vi "TDMSLoader.vi"(8 "Error in":errorcluster, 11 "Measurements path":path=path "") -> (0 "Error out":errorcluster)   [LabVIEW 2019]
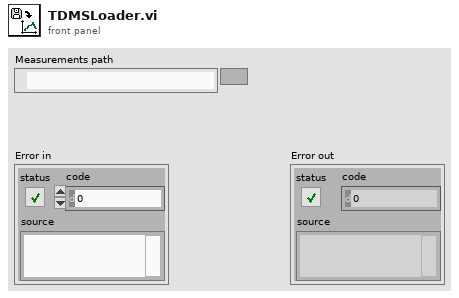
[diagram p1: front panel]
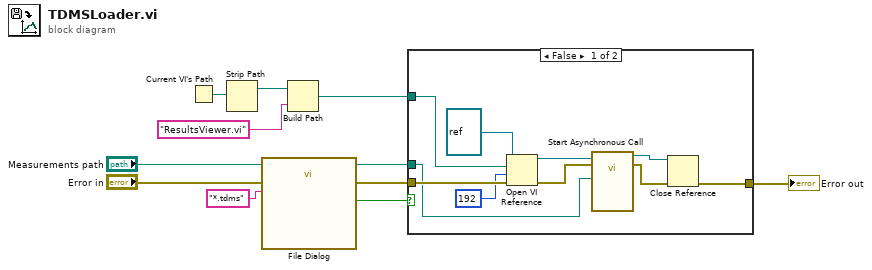
[diagram p0: block diagram]
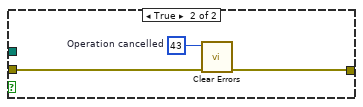
[diagram p2: hidden frame]
diagram:
  n1 = Current VI's Path() -> (path=w4:path)
  n2 = Strip Path(path=w4) -> (stripped path=w3:path)  [unwired: 1 out]
  n3 = call "File Dialog"("start path"="Measurements path", "error in"="Error in", "pattern (all files)"="*.tdms") -> ("selected path"=w10:path, "cancelled"=w6:bool, "error out"=w7:errorcluster)  [unwired: 9 in, 1 out]
  n4 = Build Path(base path=w3, name or relative path="ResultsViewer.vi" ("pattern (all files)")) -> (appended path=w1:path)
  n5 = case shown="False" w6 {
    tunnel: w7 -> [w21 w24]
    tunnel: w10 -> [w16 _]
    tunnel: [w13 w22] -> w5
    tunnel: w1 -> [w19 _]
    frame False {
      n6 = Open VI Reference(type specifier VI Refnum (for type only)=refnum<vi> refnum, vi path=w19, options=192, error in (no error)=w21) -> (vi reference=w17:refnum<vi>, error out=w15:errorcluster)  [unwired: 2 in]
      n7 = call-by-ref "Start Asynchronous Call"(reference=w17, error in=w15, "TDMS path"=w16) -> (reference out=w14:refnum<vi>, error out=w12:errorcluster)  [unwired: 10 in, 1 out]
      n8 = Close Reference(reference=w14, error in (no error)=w12) -> (error out=w13:errorcluster)
    }
    frame True {
      w23 = 43  # Operation cancelled
      n9 = call <vilib>:"Clear Errors.vi"("error in (no error)"=w24, "specific error code to clear (0: all)"=w23) -> ("error out"=w22:errorcluster)  [unwired: 4 in, 1 out]
    }
  }
  "Error out" <- w5
